vi "Describe Cluster.vi"(11 "Cluster":variant) -> (2 "Elements":string[](array[string]))   [LabVIEW 2020]
uses:
  Framework/Utilities/Utilities.lvlib
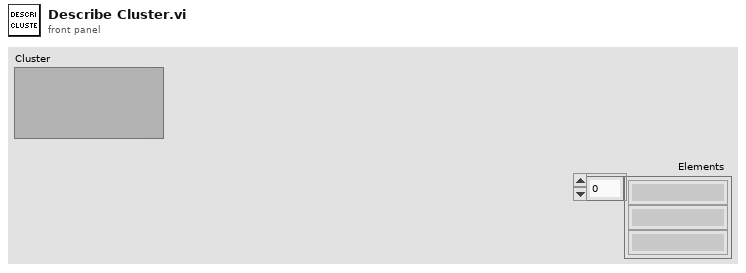
[diagram p1: front panel]
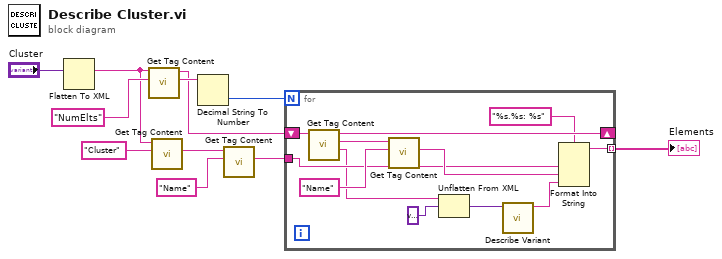
[diagram p0: block diagram]
diagram:
  n1 = Flatten To XML(6:"Cluster") -> (2:w3:string)
  n2 = call "Get Tag Content.vi"("Tag"="NumElts" ("regular expression"), "xml string in"=w3) -> ("Tag content"=w7:string, "After end of tag"=w6:string)  [unwired: 7 in, 1 out]
  n3 = call "Get Tag Content.vi"("Tag"="Cluster", "xml string in"=w3) -> ("Tag content"=w1:string)  [unwired: 7 in, 2 out]
  n4 = Decimal String To Number(string=w7) -> (number=w8:i32)  [unwired: 2 in, 1 out]
  n5 = call "Get Tag Content.vi"("Tag"="Name" ("regular expression"), "xml string in"=w1) -> ("Tag content"=w4:string)  [unwired: 7 in, 2 out]
  n6 = for {
    N: w8 -> [_]
    tunnel: [w21] -> w9 mode=indexing
    shift-right: [w22] -> _
    shift-left: w6 -> [w23]
    tunnel: w4 -> [w17]
    n7 = call "Get Tag Content.vi"("xml string in"=w23) -> ("Tag with Content"=w12:string, "Tag content"=w18:string, "After end of tag"=w22:string)  [unwired: 8 in]
    n8 = call "Get Tag Content.vi"("Tag"="Name" ("regular expression"), "xml string in"=w18) -> ("Tag content"=w19:string)  [unwired: 7 in, 2 out]
    n9 = Unflatten From XML(xml string=w12, type=variant) -> (value=w14:variant)  [unwired: 1 in, 1 out]
    n10 = call "Describe Variant.vi"("Variant"=w14) -> ("Variant Description"=w13:string)  [unwired: 8 in, 2 out]
    n11 = Format Into String(format string="%s.%s: %s", w17, w19, w13) -> (resulting string=w21:string)  [unwired: 2 in, 1 out]
  }
  "Elements" <- w9
